vi "UDP test Half 1.vi"() -> ()   [LabVIEW 2013, in "TEC tests.lvlib"]
uses:
  TEC tests.lvlib
  execution/TEC runtime.lvclass
  configuration/TEC configuration.lvclass
  <vilib>/NI/Module Timing Source/usec timing source/usec timing source.lvclass
  configuration/TEC configuration.lvclass/TEC configuration.ctl
  <vilib>/NI/Tag Bus/table/data polymorphs/write one/write Double.vi
  <vilib>/NI/Tag Bus/table/data polymorphs/write one/write Array of U64.vi
  configuration/Write receive on port.vi
  configuration/Write send from port.vi
  configuration/Write send to address.vi
  configuration/Write send to port.vi
  <vilib>/NI/Configuration Framework/serializable configuration/NISE_CEF_serializable configuration.lvclass
  <vilib>/NI/Tag Bus/table/data table.lvlib
  <vilib>/ptbypt/NI_PtbyPt.lvlib
panel:
  in  "value":u64[](array[numeric])
  out "name":string
  in  "send to address":string="NI-cRIO-9068-018CF33E"
  out "duration avg":dbl
  in  "dt":u32=100
  out "duration":dbl
  out "final":errorcluster
  in  "value tx":dbl
  in  "stop":bool
  out "init err":errorcluster
  in  "ch count":i32=100
  out "serialization problem":errorcluster
  out "invalid configuration":errorcluster
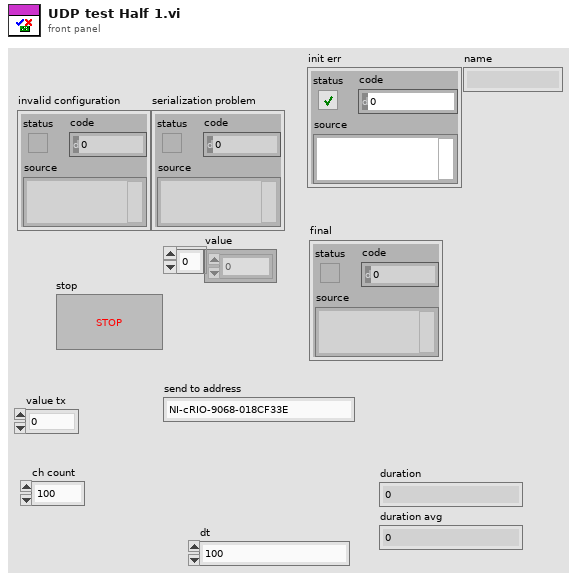
[diagram p1: front panel]
types:
  T1 = typedef "TBM channel.lvclass/data tables.ctl" = cluster{"input data":T2, "processing parameter":T2, "processing result":T2, "output data":T2}
  T2 = typedef "tag bus.lvlib/dictionary table pair.ctl" = cluster{"data dictionary":refnum<class "data dictionary.lvclass">, "data table":T3}
  T3 = typedef "tag bus.lvlib/data table.lvlib/data table.ctl" = cluster{"Double":dbl[], "Single":sgl[], "I64":i64[], "I32":i32[], "I16":i16[], "I8":i8[], "U64":u64[], "U32":u32[], "U16":u16[], "U8":u8[], "Boolean":bool[], "String":string[], "Array of Double":cluster{"DBL Array":dbl[]}[], "Array of Single":cluster{"SGL Array":sgl[]}[], "Array of I64":cluster{"I64 Array":i64[]}[], "Array of I32":cluster{"I32 Array":i32[]}[], "Array of I16":cluster{"I16 Array":i16[]}[], "Array of I8":cluster{"I8 Array":i8[]}[], "Array of U64":cluster{"U64 Array":u64[]}[], "Array of U32":cluster{"U32 Array":u32[]}[], "Array of U16":cluster{"U16 Array":u16[]}[], "Array of U8":cluster{"U8 Array":u8[]}[], "Array of Boolean":cluster{"Boolean Array":bool[]}[], "Array of String":cluster{"String Array":string[]}[]}
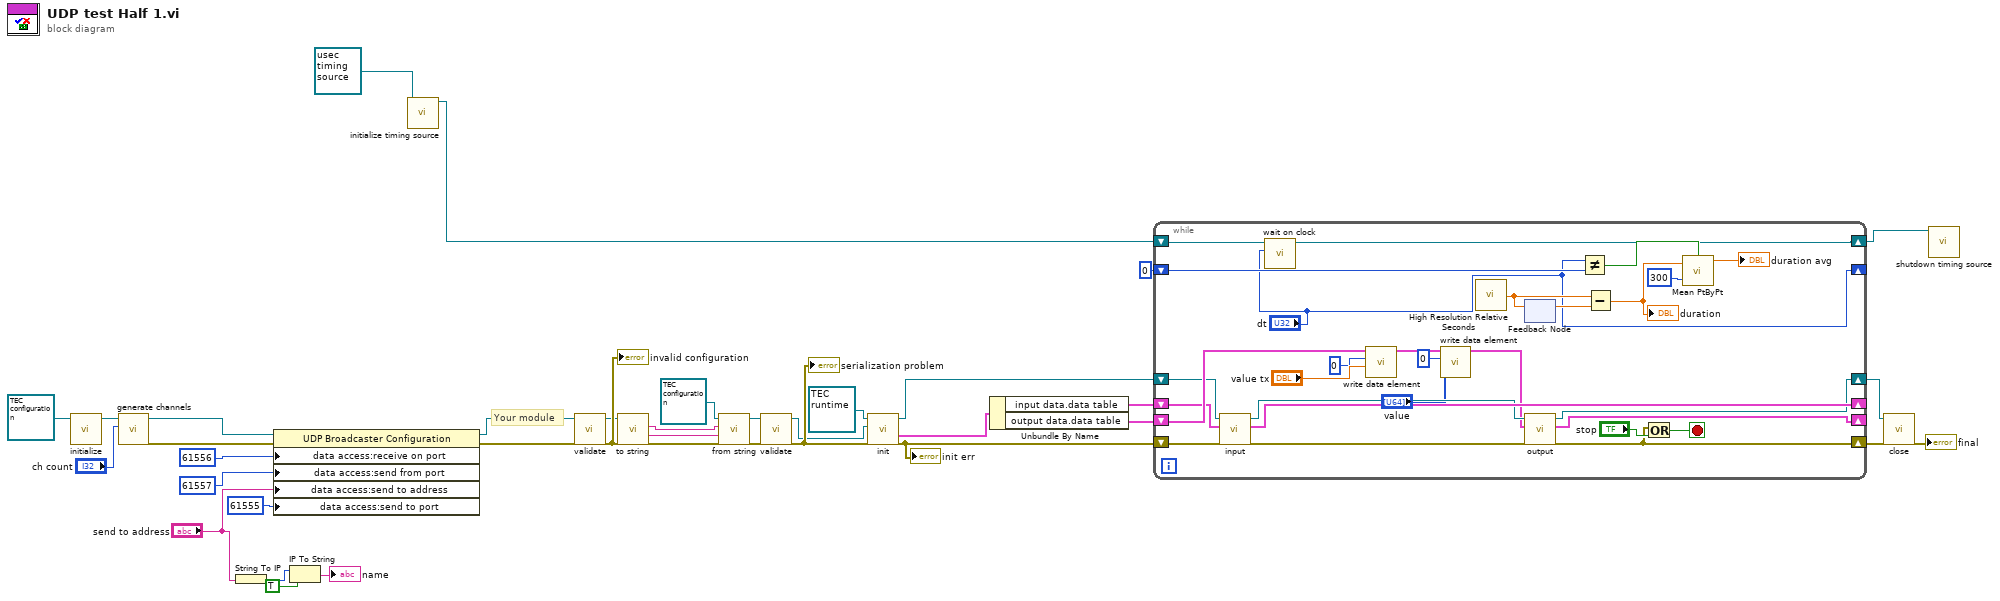
[diagram p0: block diagram]
diagram:
  # "Your module"
  n1 = call <vilib>:"initialize.vi"("configuration in"=refnum<class "TEC configuration.lvclass"> refnum ("tag bus configurable plugin module configuration")) -> ("configuration out"=w9:refnum<class "TEC configuration.lvclass">)  [unwired: 8 in, 2 out]
  n2 = call "generate channels.vi"("ch count"="ch count", "TEC configuration in"=w9) -> ("error out"=w27:errorcluster, "TEC configuration out"=w25:refnum<class "TEC configuration.lvclass">)  [unwired: 8 in]
  n3 = String To IP(1:"send to address") -> (0:w6:u32)
  n4 = property class="UDP Broadcaster Configuration"(reference=w25, error in=w27, "data access:receive on port"=u16 61556 ("send from port"), "data access:send from port"=u16 61557 ("send to port"), "data access:send to address"="send to address", "data access:send to port"=u16 61555 ("receive on port")) -> (reference out=w24:refnum<class "TEC configuration.lvclass">, error out=w26:errorcluster)
  n5 = IP To String(1:TRUE ("dot notation? (F)"), 2:w6) -> (0:→"name":string)
  n6 = call-dynamic "initialize timing source.vi"("timing source in"=refnum<class "usec timing source.lvclass"> refnum ("usec timing source.lvclass")) -> ("timing source out"=w2:refnum<class "usec timing source.lvclass">)  [unwired: 9 in, 1 out]
  n7 = call-dynamic "validate.vi"("error in"=w26, "TEC configuration in"=w24) -> ("error out"=w37:errorcluster, "TEC configuration out"=w20:refnum<class "TEC configuration.lvclass">)  [unwired: 8 in]
  "invalid configuration" <- w37
  n8 = call-dynamic "to string.vi"("error in"=w37, "TEC configuration in"=w20) -> ("error out"=w34:errorcluster, "data"=w35:string, "version"=w36:string)  [unwired: 6 in, 1 out]
  n9 = call-dynamic "from string.vi"("error in"=w34, "data"=w35, "version"=w36, "TEC configuration in"=refnum<class "TEC configuration.lvclass"> refnum) -> ("error out"=w32:errorcluster, "TEC configuration out"=w33:refnum<class "TEC configuration.lvclass">)  [unwired: 6 in]
  n10 = call-dynamic "validate.vi"("error in"=w32, "TEC configuration in"=w33) -> ("error out"=w30:errorcluster, "TEC configuration out"=w29:refnum<class "TEC configuration.lvclass">)  [unwired: 8 in]
  "serialization problem" <- w30
  n11 = call-dynamic "init.vi"("error in"=w30, "TBM module configuration in"=w29, "TEC runtime in"=refnum<class "TEC runtime.lvclass"> refnum ("tag bus configurable plugin module")) -> ("error out"=w18:errorcluster, "data allocations"=w17:T1, "TEC runtime out"=w14:refnum<class "TEC runtime.lvclass">)  [unwired: 5 in, 1 out]
  "init err" <- w18
  n12 = Unbundle By Name(w17) -> ("input data.data table"=w16:T3, "output data.data table"=w15:T3)
  n13 = while {
    shift-right: [w52] -> _
    shift-left: w15 -> [w63]
    shift-right: [w58] -> _
    shift-left: w16 -> [w59]
    shift-right: [w54] -> w11
    shift-left: w14 -> [w60]
    shift-right: [w51] -> w13
    shift-left: w18 -> [w57]
    shift-right: ["dt"] -> _
    shift-left: u32 0 ("millisecond multiple") -> [w46]
    shift-right: [w39] -> w1
    shift-left: w2 -> [w40]
    stop <- w64 stop-if-true
    n14 = call-dynamic "input.vi"("error in"=w57, "data table in"=w59, "TEC runtime in"=w60) -> ("error out"=w56:errorcluster, "data table out"=w58:T3, "TEC runtime out"=w55:refnum<class "TEC runtime.lvclass">)  [unwired: 6 in]
    n15 = call-dynamic "wait on clock.vi"("dt"="dt", "timing source in"=w40) -> ("timing source out"=w39:refnum<class "usec timing source.lvclass">)  [unwired: 7 in, 2 out]
    n16 = call-poly <vilib>:"write data element.vi"("value"="value tx", "index"=0, "data table in"=w63) -> ("data table out"=w53:T3)  [unwired: 8 in]
    n17 = call-poly <vilib>:"write data element.vi"("value"="value", "index"=0, "data table in"=w53) -> ("data table out"=w43:T3)  [unwired: 8 in]
    n18 = call <vilib>:"High Resolution Relative Seconds.vi"() -> ("relative seconds"=w49:dbl)
    n19 = feedback-in #1(w49) -> ()
    n20 = feedback #1() -> (w50:dbl)  [unwired: 1 in]
    n21 = call-dynamic "output.vi"("error in"=w56, "data table in"=w43, "TEC runtime in"=w55) -> ("error out"=w51:errorcluster, "data table out"=w52:T3, "TEC runtime out"=w54:refnum<class "TEC runtime.lvclass">)  [unwired: 6 in]
    n22 = Not Equal?(x="dt", y=w46) -> (x != y?=w45:bool)
    n23 = Subtract(x=w49, y=w50) -> (x-y=w48:dbl)
    "duration" <- w48
    n24 = Or(x=w51, y="stop") -> (x .or. y?=w64:bool)
    n25 = call <vilib>:"Mean PtByPt.vi"("x"=w48, "sample length"=300, "initialize"=w45) -> ("mean"=→"duration avg":dbl)  [unwired: 1 in, 1 out]
  }
  n26 = call-dynamic "close.vi"("error in"=w13, "TEC runtime in"=w11) -> ("error out"=→"final":errorcluster)  [unwired: 9 in]
  n27 = call-dynamic "shutdown timing source.vi"("timing source in"=w1) -> ()  [unwired: 9 in, 2 out]
